vi "Automatic Motor Controller.vi"(8 "Speed":dbl(slide) scale=0.0..1.0, 9 "Right":bool, 10 "Left":bool, 11 "Forward":bool) -> (0 "Duty Cycle B2":dbl, 1 "Duty Cycle B1":dbl, 2 "Duty Cycle A2":dbl, 3 "Duty Cycle A1":dbl)   [LabVIEW 2019]
doc: "The motor controlling programmation for the Automatic Drive.\nInputs Forward, Left, Right are booleans to indicate in which direction you would like to drive.\nInput Speed is to limit the speed at which the motors will turn."
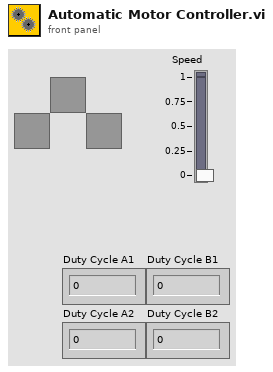
[diagram p1: front panel]
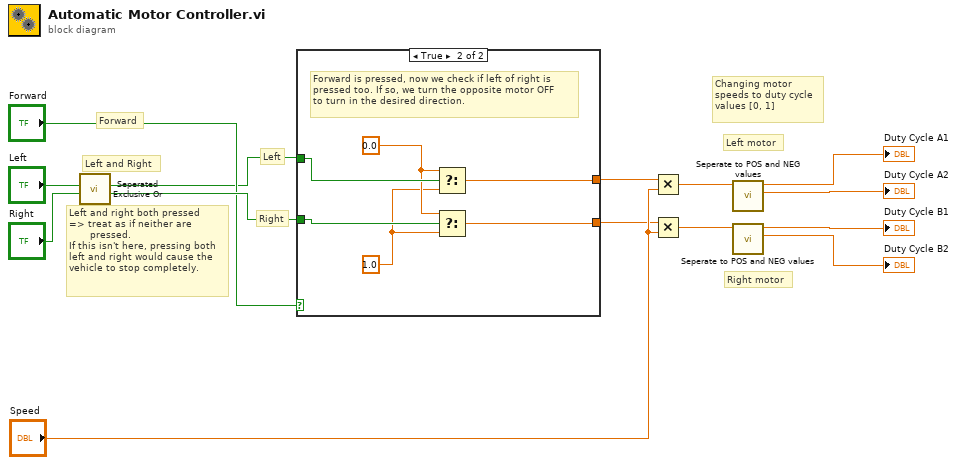
[diagram p0: block diagram]
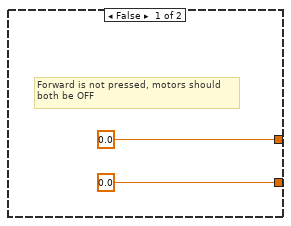
[diagram p2: hidden frame]
diagram:
  # "Right"
  # "Left"
  # "Left and right both pressed\n=> treat as if neither are\n       pressed.\nIf this isn't here, pressing both\nleft and right would cause the\nvehicle to stop completely."
  # "Changing motor\nspeeds to duty cycle\nvalues [0, 1]"
  # "Right motor"
  # "Left motor"
  # "Left and Right"
  # "Forward"
  n1 = call "Seperated Exclusive Or.vi"("q"="Right", "p"="Left") -> ("only q"=w5:bool, "only p"=w3:bool)  [unwired: 8 in]
  n2 = case shown="True" "Forward" {
    tunnel: w5 -> [_ w19]
    tunnel: w3 -> [_ w20]
    tunnel: [0.0 w22] -> w2
    tunnel: [0.0 w21] -> w1
    frame False {
      # "Forward is not pressed, motors should\nboth be OFF"
    }
    frame True {
      w18 = 0.0 ("Curving\nFactor")
      w17 = 1.0
      # "Forward is pressed, now we check if left of right is\npressed too. If so, we turn the opposite motor OFF\nto turn in the desired direction."
      n3 = Select(t=w18, s=w20, f=w17) -> (s? t:f=w22:dbl)
      n4 = Select(t=w18, s=w19, f=w17) -> (s? t:f=w21:dbl)
    }
  }
  n5 = Multiply(x=w2, y="Speed") -> (x*y=w11:dbl)
  n6 = Multiply(x=w1, y="Speed") -> (x*y=w10:dbl)
  n7 = call "Seperate to POS and NEG values.vi"("Motorspeed"=w11) -> ("Duty Cycle 2"=→"Duty Cycle A2":dbl, "Duty Cycle 1"=→"Duty Cycle A1":dbl)  [unwired: 9 in]
  n8 = call "Seperate to POS and NEG values.vi"("Motorspeed"=w10) -> ("Duty Cycle 2"=→"Duty Cycle B2":dbl, "Duty Cycle 1"=→"Duty Cycle B1":dbl)  [unwired: 9 in]
